vi "Create from VI.vi"(8 "error in (no error)":errorcluster, 9 "Test Method VI Path":path, 10 "Test Case LVCLass Path":path) -> (0 "error out":errorcluster, 3 "LUnit Test Case Out":refnum<class "LUnit Test Case.lvclass">)   [LabVIEW 2020, in "LUnit Test Case.lvclass"]
uses:
  LUnit Test Case.lvclass
  LUnit Test Case.lvclass/LUnit Test Case.ctl
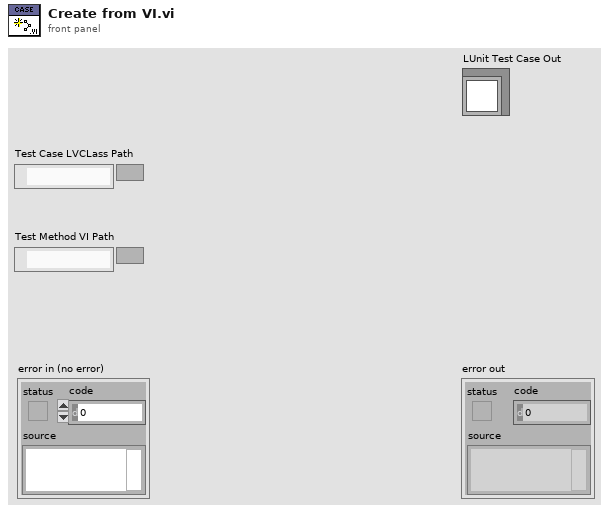
[diagram p1: front panel]
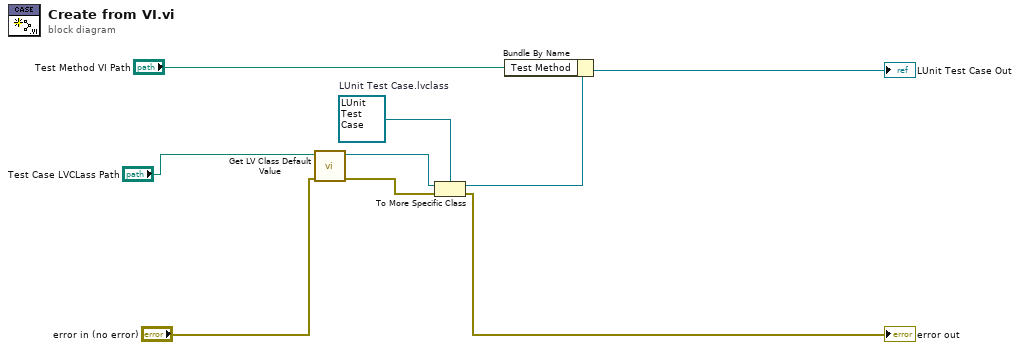
[diagram p0: block diagram]
diagram:
  w1 = refnum<class "LUnit Test Case.lvclass"> refnum  # LUnit Test Case.lvclass
  n1 = call <vilib>:"Get LV Class Default Value.vi"("error in (no error)"="error in (no error)", "class path"="Test Case LVCLass Path") -> ("error out"=w5:errorcluster, "object"=w6:refnum<class>)  [unwired: 8 in]
  n2 = To More Specific Class(target class=w1, reference=w6, error in=w5) -> (specific class reference=w7:refnum<class "LUnit Test Case.lvclass">, error out=→"error out":errorcluster)
  n3 = Bundle By Name(cluster=w7, "Test Method"="Test Method VI Path") -> (→"LUnit Test Case Out":refnum<class "LUnit Test Case.lvclass">)
